vi "Peak Density Check if Point Exists in Array.vi"(2 "Point":T1, 3 "Array":T1[](array[typedef])) -> (0 "Exists?":bool, 1 "Index":i32)   [LabVIEW 2018, in "Video Cam Processor.lvclass"]
uses:
  Video Cam Processor.lvclass
  Private/Hull Point STYP.ctl
  d1ab6953-b824-47f1-af91-2b71ef3c3e57.vi
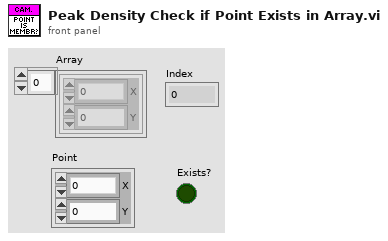
[diagram p1: front panel]
types:
  T1 = typedef "Video Cam Processor.lvclass/Hull Point STYP.ctl" = cluster{"X":i32, "Y":i32}
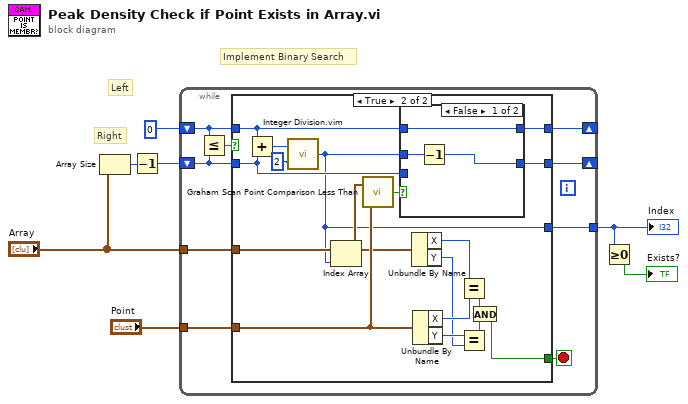
[diagram p0: block diagram]
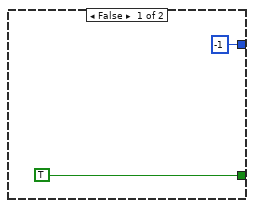
[diagram p2: hidden frame]
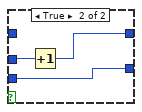
[diagram p3: hidden frame]
diagram:
  # "Right"
  # "Left"
  # "Implement Binary Search"
  n1 = Array Size(array="Array") -> (size(s)=w5:i32)
  n2 = Decrement(x=w5) -> (x-1=w4:i32)
  n3 = while {
    tunnel: "Array" -> [w15]
    tunnel: "Point" -> [w14]
    shift-right: [w9] -> _
    shift-left: w4 -> [w11]
    shift-right: [w10] -> _
    shift-left: 0 -> [w12]
    tunnel: [w8] -> w1
    stop <- w16 stop-if-true
    n4 = Less Or Equal?(x=w12, y=w11) -> (x <= y?=w13:bool)
    n5 = case shown="True" w13 {
      tunnel: [TRUE w30] -> w16
      tunnel: w15 -> [_ w21]
      tunnel: w14 -> [_ w29]
      tunnel: w12 -> [_ w26]
      tunnel: w11 -> [_ w24]
      tunnel: [_ w23] -> w10
      tunnel: [_ w22] -> w9
      tunnel: [-1 ("X // Y") w19] -> w8
      frame False {
      }
      frame True {
        n6 = Add(x=w26, y=w24) -> (x+y=w27:i32)
        n7 = call "Integer Division.vim"("Y"=2, "X"=w27) -> ("X // Y"=w19:i32)
        n8 = Index Array(array=w21, index=w19) -> (element=w20:T1)
        n9 = call "Graham Scan Point Comparison Less Than.vi"("B"=w29, "A"=w20) -> ("A < B?"=w25:bool)
        n10 = case shown="False" w25 {
          tunnel: w26 -> [w39 _]
          tunnel: w24 -> [_ w40]
          tunnel: w19 -> [w38 w42]
          tunnel: [w39 w41] -> w23
          tunnel: [w37 w40] -> w22
          frame False {
            n11 = Decrement(x=w38) -> (x-1=w37:i32)
          }
          frame True {
            n12 = Increment(x=w42) -> (x+1=w41:i32)
          }
        }
        n13 = Unbundle By Name(w20) -> ("X"=w36:i32, "Y"=w33:i32)
        n14 = Unbundle By Name(w29) -> ("X"=w35:i32, "Y"=w34:i32)
        n15 = Equal?(x=w35, y=w36) -> (x = y?=w31:bool)
        n16 = Equal?(x=w34, y=w33) -> (x = y?=w32:bool)
        n17 = And(x=w31, y=w32) -> (x .and. y?=w30:bool)
      }
    }
  }
  "Index" <- w1
  n18 = Greater Or Equal To 0?(x=w1) -> (x >= 0?=→"Exists?":bool)
